vi "DIO Bit Write.vi"(0 "DIO Device":tag, 1 "Wait (ms)":u32=50, 5 "Port":string, 7 "Line":string, 9 "On/Off":bool, 11 "error in (no error)":errorcluster) -> (15 "error out":errorcluster)   [LabVIEW 2025, in "niMIO.lvclass"]
uses:
  niMIO.lvclass
  <vilib>/DAQmx/write.llb/DAQmx Write (Digital Bool 1Line 1Point).vi
  <vilib>/DAQmx/create/channels.llb/DAQmx Create Channel (DO-Digital Output).vi
  <vilib>/DAQmx/miscellaneous.llb/DAQmx Fill In Error Info.vi
  niMIO.lvclass/niMIO.ctl
panel:
  out "niDIO out":refnum<class "niMIO.lvclass">
  in  "niDIO in":refnum<class "niMIO.lvclass">
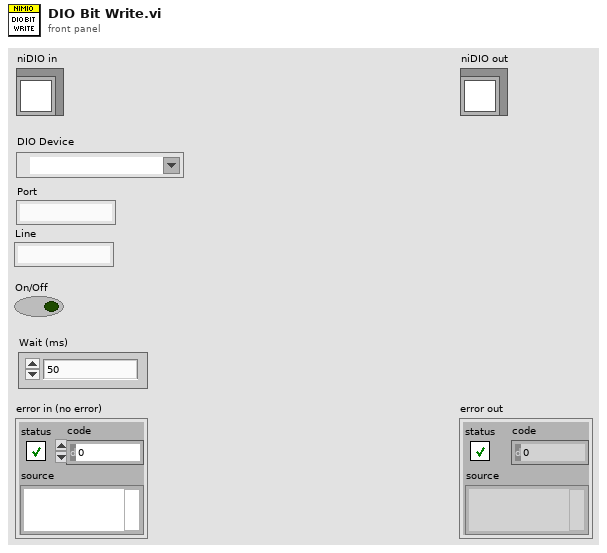
[diagram p1: front panel]
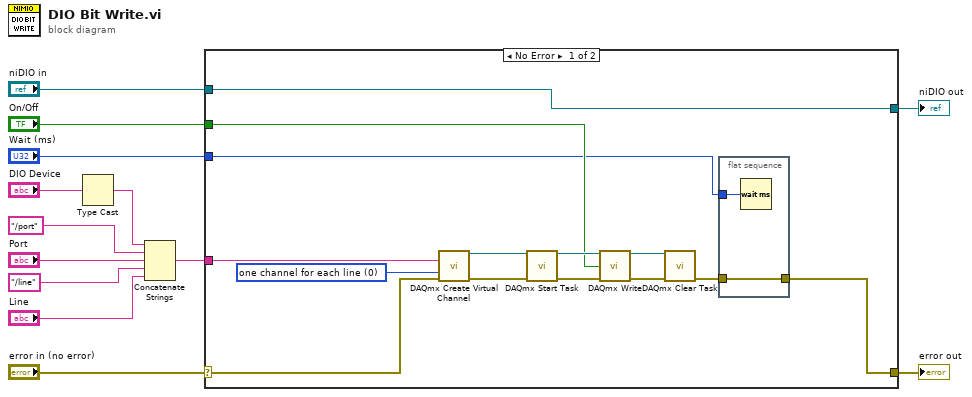
[diagram p0: block diagram]
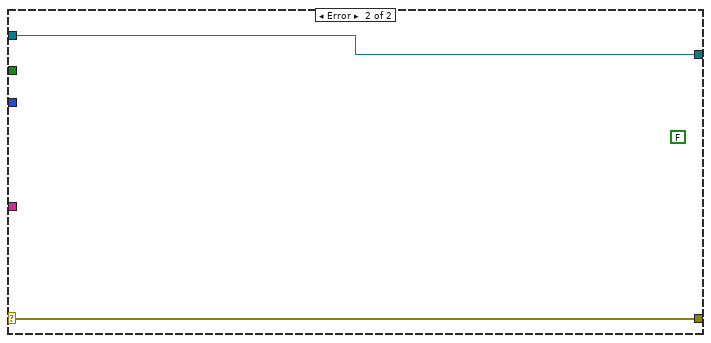
[diagram p2: hidden frame]
diagram:
  n1 = Type Cast(x="DIO Device") -> (*(type *) &x=w6:string)  [unwired: 1 in]
  n2 = Concatenate Strings(w6, "/port", "Port", "/line" ("string"), "Line") -> (w4:string)
  n3 = case shown="No Error" "error in (no error)" {
    selector: "error in (no error)" -> [w18 w31]
    tunnel: [w15 w31] -> w12
    tunnel: [w27 w30] -> w10
    tunnel: "niDIO in" -> [w27 w30]
    tunnel: w4 -> [w19 _]
    tunnel: "On/Off" -> [w17 _]
    tunnel: "Wait (ms)" -> [w14 _]
    frame No Error {
      w24 = 0 items=["one channel for each line", "one channel for all lines"] ("line grouping")
      n4 = call-poly <vilib>:"DAQmx Create Virtual Channel.vi"("lines"=w19, "line grouping"=w24, "error in"=w18) -> ("task out"=w26:refnum<k21>, "error out"=w25:errorcluster)  [unwired: 11 in]
      n5 = call <vilib>:"DAQmx Start Task.vi"("task/channels in"=w26, "error in"=w25) -> ("task out"=w23:refnum<k21>, "error out"=w22:errorcluster)  [unwired: 12 in]
      n6 = call-poly <vilib>:"DAQmx Write.vi"("task/channels in"=w23, "data"=w17, "error in"=w22) -> ("task out"=w21:refnum<k21>, "error out"=w20:errorcluster)  [unwired: 10 in, 1 out]
      n7 = call <vilib>:"DAQmx Clear Task.vi"("task in"=w21, "error in"=w20) -> ("error out"=w16:errorcluster)  [unwired: 13 in]
      n8 = flat-sequence {
        tunnel: w16 -> [w28]
        tunnel: [w28] -> w15
        tunnel: w14 -> [w29]
        frame #0 {
          n9 = Wait (ms)(milliseconds to wait=w29) -> ()  [unwired: 1 out]
        }
      }
    }
    frame Error {
      (unwired) FALSE ("data")
    }
  }
  "error out" <- w12
  "niDIO out" <- w10
